vi "Untitled 3.vi"() -> ()   [LabVIEW 2012]
panel:
  in  "ПУ":bool
  out "к MUX":bool
  out "упр для MUX и МВВ":bool
  in  "КК2":bool
  in  "КК1":bool
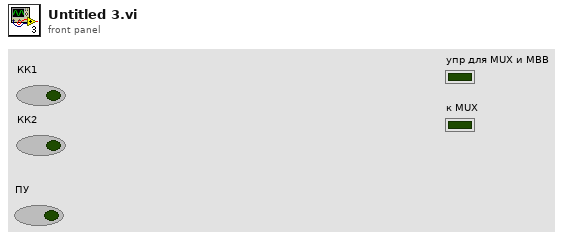
[diagram p1: front panel]
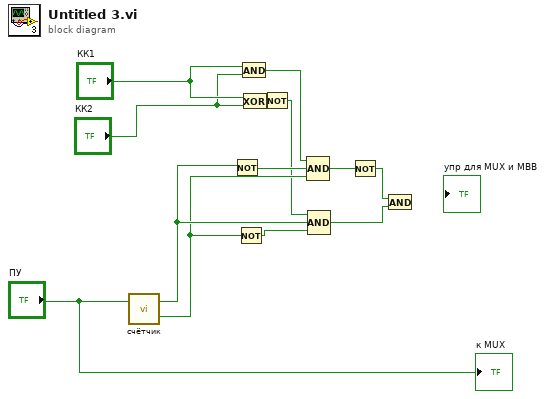
[diagram p0: block diagram]
diagram:
  n1 = call "счётчик.vi"("T"="ПУ") -> ("x1"=w9:bool, "x0"=w10:bool)  [unwired: 1 in]
  n2 = Not(x=w10) -> (.not. x?=w12:bool)
  n3 = Not(x=w9) -> (.not. x?=w11:bool)
  n4 = And(x="КК1", y="КК2") -> (x .and. y?=w13:bool)
  n5 = Exclusive Or(1:"КК2", 2:"КК1") -> (0:w6:bool)
  n6 = Not(x=w6) -> (.not. x?=w5:bool)
  n7 = Compound Arithmetic op=AND(w13, w12, w9) -> (w3:bool)
  n8 = Compound Arithmetic op=AND(w5, w10, w11) -> (w1:bool)
  n9 = Not(x=w3) -> (.not. x?=w2:bool)
  n10 = And(x=w2, y=w1) -> ()  [unwired: 1 out]
  "к MUX" <- "ПУ"
